vi "PC VI 2.vi"() -> ()   [LabVIEW 2023]
uses:
  <vilib>/rvi/interface/nirviOpenFPGA/nirviOpenFPGA.xnode
  <vilib>/rvi/interface/nirviMethod/nirviMethod.xnode
  <vilib>/rvi/errors/niLvFpgaMergeErrorWithErrorCode.vi
  <vilib>/FPGAPlugInAG/Dynamic/niLvFpga_Run_Dynamic.vi
  <vilib>/rvi/interface/nirviReadWriteControl/nirviReadWriteControl.xnode
  <vilib>/rvi/interface/nirviCloseFPGA/nirviCloseFPGA.xnode
  <vilib>/express/express shared/transition.llb/Dynamic To Waveform Array.vi
  <vilib>/express/express signal manip/GetorSetDDTAttributes/Set DDT Attributes/SetT0.vi
  <vilib>/express/express shared/transition.llb/Waveform Array To Dynamic.vi
  <vilib>/express/express signal manip/GetorSetDDTAttributes/Set DDT Attributes/Set DDT Properties.xnode
  FPGA Bitfiles/wip_FPGATarget_FPGAVIwithFFT_RH-sP0Zqczc.lvbitx
  FPGA VI with RMS.vi
  <vilib>/FPGAPlugInAG/USB-7856R OEM/niLvFpga_Open_USB-7856R OEM.vi
  <vilib>/rvi/interface/common/dynamic/niFpgaDynamicAddResources.vi
  <vilib>/FPGAPlugInAG/Dynamic/niLvFpga_ConfigureFifo_Dynamic.vi
  <vilib>/FPGAPlugInAG/Dynamic/niLvFpga_StartFifo_Dynamic.vi
  NiFpgaLv.dll
  <vilib>/Utility/error.llb/Error Cluster From Error Code.vi
  <vilib>/rvi/interface/Simulation/niFpgaSimulationCallBeginRW.vi
  <vilib>/rvi/errors/niLvFpgaAdjustHostInterfaceError.vi
  <vilib>/FPGAPlugInAG/Dynamic/niLvFpga_ReadFifo_Dynamic.vi
  <vilib>/FPGAPlugInAG/Dynamic/niLvFpga_Close_Dynamic.vi
panel:
  out "Elements Remaining":u32
  out "current frequency":dbl
  out "Waveform Chart":sgl[](graph)
  in  "Step Value":dbl=5.0
  out "Number of steps":dbl=nan
  in  "Starting frequency":dbl=32700.0
  in  "Ending frequency":dbl=32800.0
  out "Actual Depth":u32
  out "Timed Out?":bool
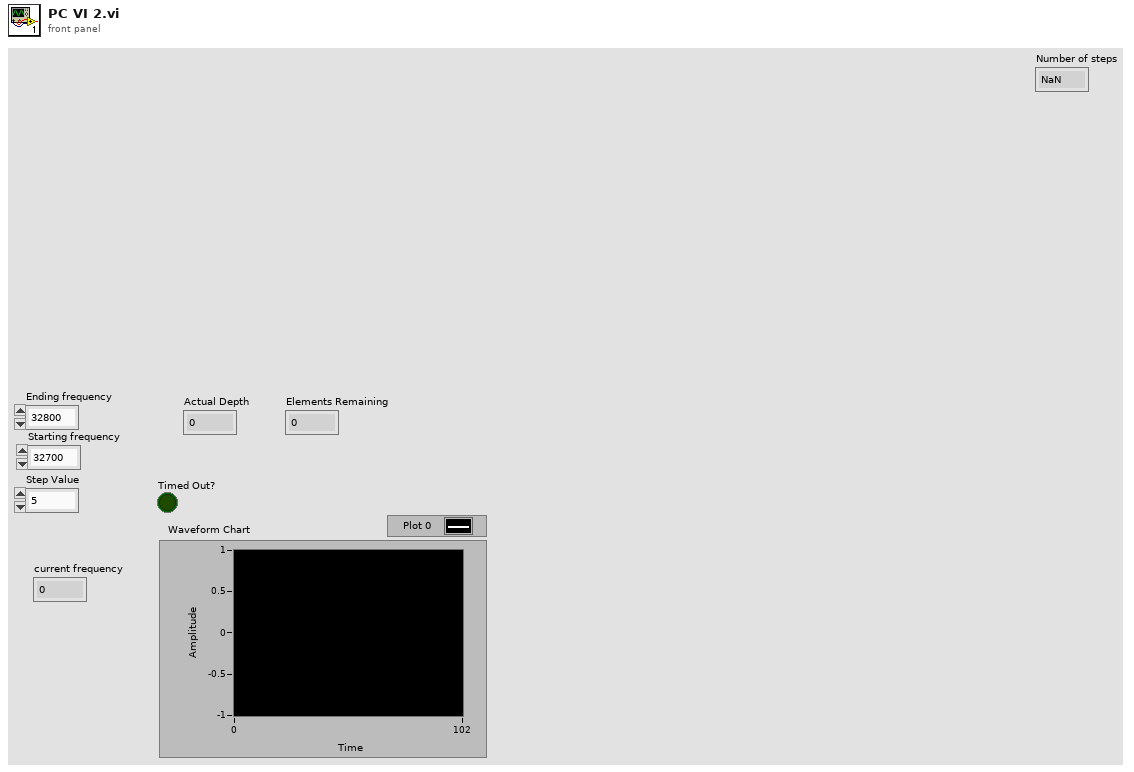
[diagram p1: front panel]
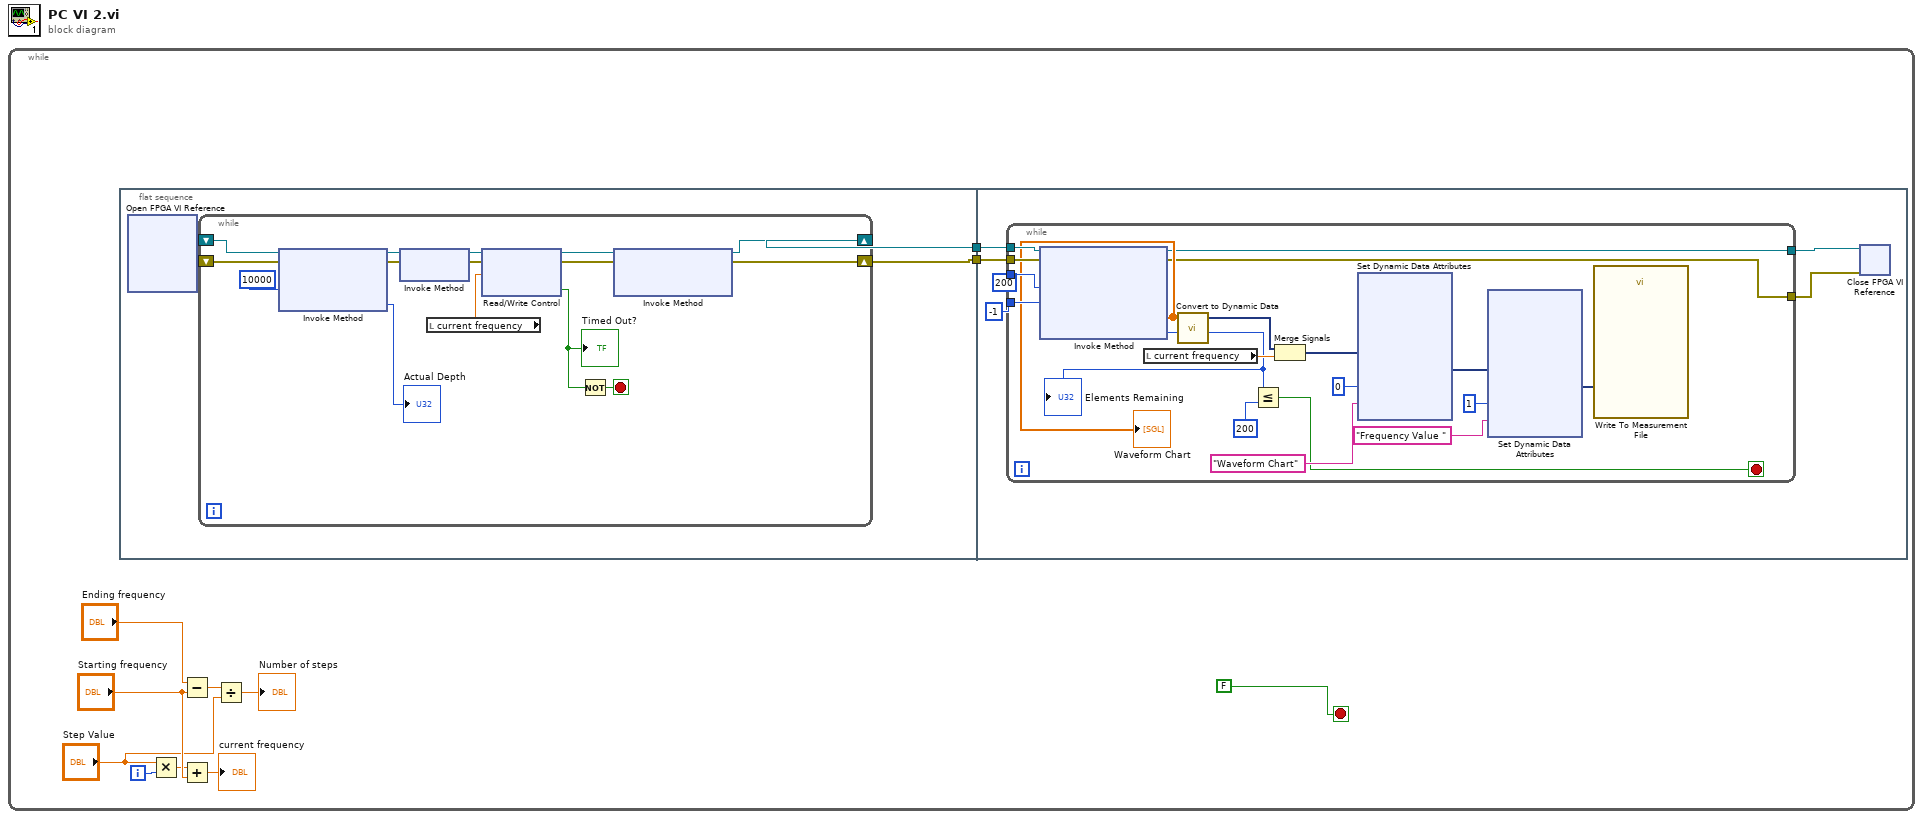
[diagram p0: block diagram]
diagram:
  n1 = while {
    i -> [w1]
    stop <- FALSE stop-if-true
    n2 = flat-sequence {
      tunnel: [w13] -> w11
      tunnel: [w12] -> w10
      tunnel: w11 -> [w36]
      tunnel: w10 -> [w35]
      frame #0 {
        n3 = xnode "Open FPGA VI Reference"() -> ("FPGA VI Reference Out"=w14:refnum<k20>, "error out"=w15:errorcluster)  [unwired: 2 in]
        n4 = while {
          shift-right: [w19] -> w12
          shift-left: w15 -> [w25]
          shift-right: [w20] -> w13
          shift-left: w14 -> [w24]
          stop <- w16 stop-if-true
          n5 = xnode "Invoke Method"("FPGA VI Reference In"=w24, "error in"=w25, "Requested Depth"=u32 10000) -> ("FPGA VI Reference Out"=w27:refnum<k20>, "error out"=w28:errorcluster, "Actual Depth"=→"Actual Depth":u32)
          n6 = xnode "Invoke Method"("FPGA VI Reference In"=w27, "error in"=w28) -> ("FPGA VI Reference Out"=w29:refnum<k20>, "error out"=w30:errorcluster)
          n7 = local read "current frequency"() -> (w18:dbl)
          n8 = xnode "Read/Write Control"("FPGA VI Reference In"=w29, "error in"=w30, "Frequency"=w18) -> ("FPGA VI Reference Out"=w22:refnum<k20>, "error out"=w21:errorcluster, "Timed Out?"=w17:bool)
          "Timed Out?" <- w17
          n9 = Not(x=w17) -> (.not. x?=w16:bool)
          n10 = xnode "Invoke Method"("FPGA VI Reference In"=w22, "error in"=w21) -> ("FPGA VI Reference Out"=w20:refnum<k20>, "error out"=w19:errorcluster)  [unwired: 1 in]
        }
      }
      frame #1 {
        n11 = while {
          tunnel: w36 -> [w46]
          tunnel: w35 -> [w45]
          tunnel: u32 200 ("Number of Elements") -> [w44]
          tunnel: -1 ("Timeout (ms)") -> [w43]
          tunnel: [w38] -> w32
          tunnel: [w37] -> w31
          stop <- w40 stop-if-true
          n12 = xnode "Invoke Method"("FPGA VI Reference In"=w46, "error in"=w45, "Number of Elements"=w44, "Timeout (ms)"=w43) -> ("FPGA VI Reference Out"=w38:refnum<k20>, "error out"=w37:errorcluster, "Data"=w42:sgl[], "Elements Remaining"=w39:u32)
          "Waveform Chart" <- w42
          "Elements Remaining" <- w39
          n13 = local read "current frequency"() -> (w54:dbl)
          n14 = call "Convert to Dynamic Data"("Array"=w42) -> ("Dynamic Data Type"=w55:dynamicdata)  [unwired: 3 in]
          n15 = Less Or Equal?(x=w39, y=u32 200) -> (x <= y?=w40:bool)
          n16 = Merge Signals(w55, w54) -> (w53:dynamicdata)
          n17 = xnode "Set Dynamic Data Attributes"("Signals In"=w53, "Signal Index"=0, "Signal Name"="Waveform Chart") -> ("Signals Out"=w52:dynamicdata)  [unwired: 1 in, 1 out]
          n18 = xnode "Set Dynamic Data Attributes"("Signals In"=w52, "Signal Index"=1, "Signal Name"="Frequency Value ") -> ("Signals Out"=w47:dynamicdata)  [unwired: 1 in, 1 out]
          n19 = call "Write To Measurement File"("Signals"=w47) -> ()  [unwired: 16 in, 3 out]
        }
        n20 = xnode "Close FPGA VI Reference"("FPGA VI Reference In"=w32, "error in"=w31) -> ()  [unwired: 1 out]
      }
    }
    n21 = Multiply(x="Step Value", y=w1) -> (x*y=w4:dbl)
    n22 = Subtract(x="Ending frequency", y="Starting frequency") -> (x-y=w8:dbl)
    n23 = Add(x=w4, y="Starting frequency") -> (x+y=→"current frequency":dbl)
    n24 = Divide(x=w8, y="Step Value") -> (x/y=→"Number of steps":dbl)
  }
